vi "six0.vi"(5 "Boolean":bool, 8 "error in (no error)":errorcluster, 9 "byte order (0:big-endian, network order)":T1(ring), 10 "Numeric":sgl, 11 "Byte Stream File in":refnum<file>) -> (0 "error out":errorcluster, 3 "Byte Stream File out":refnum<file>)   [LabVIEW 2013]
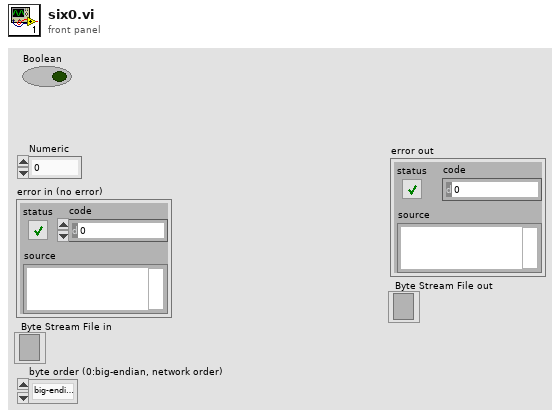
[diagram p1: front panel]
types:
  T1 = enum16{"big-endian, network order", "native, host order", "little-endian"}
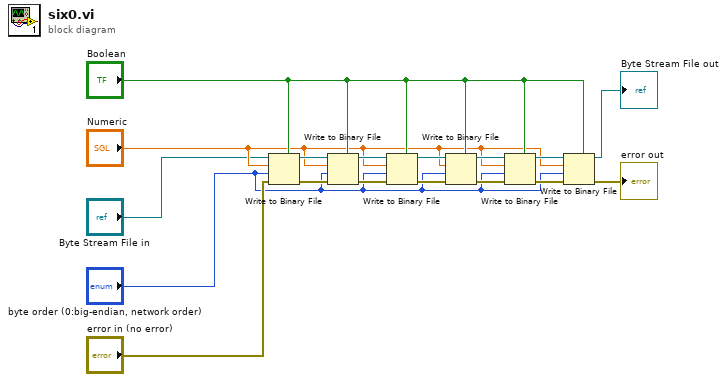
[diagram p0: block diagram]
diagram:
  n1 = Write to Binary File(file (use dialog)="Byte Stream File in", data="Numeric", error in="error in (no error)", 5:"Boolean", 9:"byte order (0:big-endian, network order)") -> (refnum out=w12:refnum<file>, error out=w17:errorcluster)  [unwired: 1 in, 1 out]
  n2 = Write to Binary File(file (use dialog)=w12, data="Numeric", error in=w17, 5:"Boolean", 9:"byte order (0:big-endian, network order)") -> (refnum out=w11:refnum<file>, error out=w16:errorcluster)  [unwired: 1 in, 1 out]
  n3 = Write to Binary File(file (use dialog)=w11, data="Numeric", error in=w16, 5:"Boolean", 9:"byte order (0:big-endian, network order)") -> (refnum out=w10:refnum<file>, error out=w15:errorcluster)  [unwired: 1 in, 1 out]
  n4 = Write to Binary File(file (use dialog)=w10, data="Numeric", error in=w15, 5:"Boolean", 9:"byte order (0:big-endian, network order)") -> (refnum out=w9:refnum<file>, error out=w14:errorcluster)  [unwired: 1 in, 1 out]
  n5 = Write to Binary File(file (use dialog)=w9, data="Numeric", error in=w14, 5:"Boolean", 9:"byte order (0:big-endian, network order)") -> (refnum out=w8:refnum<file>, error out=w13:errorcluster)  [unwired: 1 in, 1 out]
  n6 = Write to Binary File(file (use dialog)=w8, data="Numeric", error in=w13, 5:"Boolean", 9:"byte order (0:big-endian, network order)") -> (refnum out=→"Byte Stream File out":refnum<file>, error out=→"error out":errorcluster)  [unwired: 1 in, 1 out]
